vi "_PC_MS_SubVI writeToTDMS.vi"(5 "MS.Pause":refnum<vi>, 7 "warning sign":refnum<vi>, 8 "error in (no error)":errorcluster, 11 "Stop":refnum<vi>) -> (0 "error out":errorcluster)   [LabVIEW 2018]
uses:
  <vilib>/Platform/TimedLoop/XDataNode/timing_clust.ctl
  <vilib>/Platform/TimedLoop/XDataNode/nitl_modes.ctl
  <vilib>/Platform/TimedLoop/XDataNode/wakeup.ctl
  PublicSubVI/Class/FileManager/FM/ctl/_PC_Pub_FM stateMachineEnum.ctl
  PublicSubVI/Class/FileManager/FM/ctl/_PC_Pub_FM ctrlFileRefnumEnum.ctl
  <vilib>/Platform/TimedLoop/XDataNode/XDataNode.xnode
  PublicSubVI/Class/FileManager/FM.lvclass
  <vilib>/Platform/TimedLoop/XDataNode/XDNodeRunTimeDep.lvlib
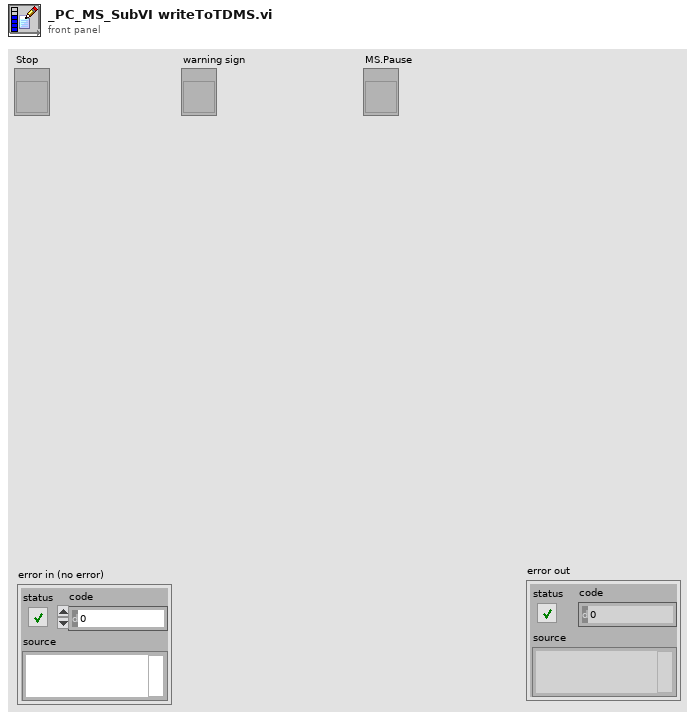
[diagram p1: front panel]
types:
  T1 = typedef "XDNodeRunTimeDep.lvlib/timing_clust.ctl" = cluster{"Expected End [f-1]":u64, "Actual End [f-1]":u64, "Finished Late? [f-1]":bool, "Expected End [i-1]":u64, "Actual End [i-1]":u64, "Finished Late? [i-1]":bool, "Expected Start [i]":u64, "Actual Start [i]":u64, "Expected Start [f]":u64, "Actual Start [f]":u64, "Source Name":string, "Structure Name":string, "Period":i64, "Deadline":i64, "Offset":i64, "Start":i64, "Priority":i32, "Timeout":i32, "Mode":T2, "Wakeup Reason":T3, "Error":errorcluster, "Source Type":string, "Secondary Source Type":string, "Global End Time":u64, "Global Start Time":u64, "Frame Duration":u64, "Iteration Duration":u64, "Assigned CPU":i32, "I/O Scan Engine Mode":u32}
  T2 = typedef "XDNodeRunTimeDep.lvlib/nitl_modes.ctl" = enum32{"No Change", "Process missed periods, maintain original phase", "Discard missed periods, maintain original phase", "Process missed periods, ignore original phase", "Discard missed periods, ignore original phase"}
  T3 = typedef "XDNodeRunTimeDep.lvlib/wakeup.ctl" = enum32{"Normal", "Aborted", "Asynchronous wakeup", "Timing source error", "Timed loop error", "Timeout"}
  T4 = enum16{"None", "Init", "Write", "Read", "PauseRead", "FinishCheck"}
  T5 = typedef "_PC_Pub_FM ctrlFileRefnumEnum.ctl" = enum16{"init", "checkFileName", "updFileName", "updWorkFolder", "updDataItems", "addNewFileName", "addSerialNum"}
  T6 = typedef "_PC_Pub_FM stateMachineEnum.ctl" = enum16{"none", "init", "reset_t0", "openTDMS", "writeTDMS", "closeTDMS", "readTDMS", "getDataItems"}
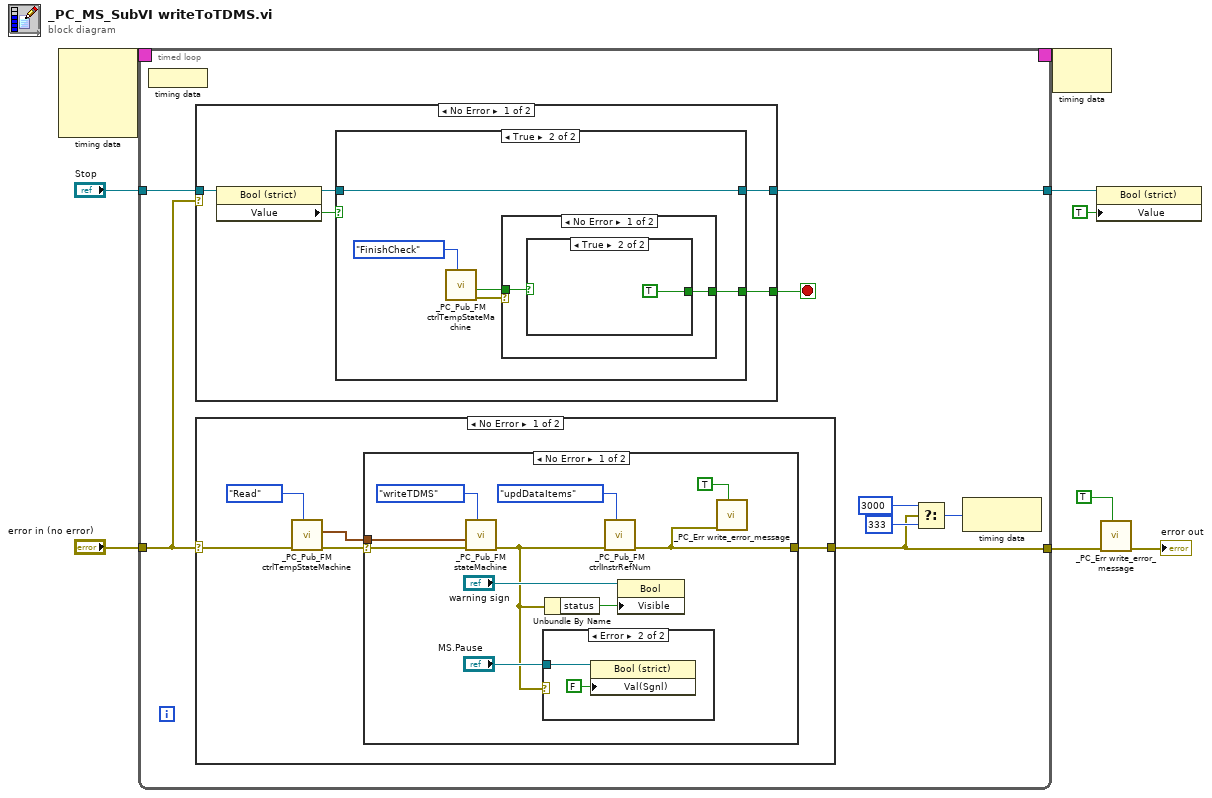
[diagram p0: block diagram]
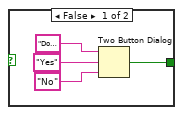
[diagram p3: hidden frame]
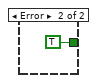
[diagram p4: hidden frame]
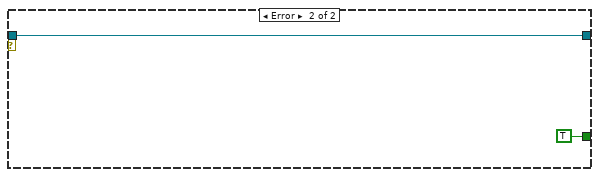
[diagram p5: hidden frame]
diagram:
  n1 = node-c288() -> (w7:T1)  [unwired: 4 in]
  n2 = timed-loop {
    tunnel: "Stop" -> [w12]
    timing: w7 -> [_]
    timing-out: [_] -> w6
    tunnel: "error in (no error)" -> [w13]
    tunnel: [w14] -> w3
    tunnel: [w11] -> w1
    stop <- w10 stop-if-true
    n3 = node-c288() -> ()  [unwired: 1 in]
    n4 = case shown="No Error" w13 {
      tunnel: [w19 TRUE] -> w10
      tunnel: w12 -> [w22 w37]
      tunnel: [w18 w37] -> w11
      frame No Error {
        n5 = property class="Bool (strict)"(reference=w22) -> (reference out=w20:refnum<vi>, "Value"=w21:bool)  [unwired: 1 in, 1 out]
        n6 = case shown="True" w21 {
          tunnel: w20 -> [w23 w24]
          tunnel: [_ w26] -> w19
          tunnel: [w23 w24] -> w18
          frame False {
          }
          frame True {
            n7 = call "_PC_Pub_FM ctrlTempStateMachine.vi"("function"=T4."FinishCheck") -> ("error out"=w25:errorcluster, "finish? (F)"=w27:bool)  [unwired: 8 in, 1 out]
            n8 = case shown="No Error" w25 {
              tunnel: w27 -> [w30 _]
              tunnel: [w29 TRUE ("T button?")] -> w26
              frame No Error {
                n9 = case shown="True" w30 {
                  tunnel: [w33 TRUE] -> w29
                  frame False {
                    n10 = Two Button Dialog(message="Do you want to interrupt this access process?", 1:"No" ("F button name (\"Cancel\")"), 2:"Yes" ("T button name (\"OK\")")) -> (T button?=w33:bool)
                  }
                  frame True {
                  }
                }
              }
              frame Error {
              }
            }
          }
        }
      }
      frame Error {
      }
    }
    n11 = case shown="No Error" w13 {
      selector: w13 -> [w42 w57]
      tunnel: [w43 w57] -> w14
      frame No Error {
        n12 = call "_PC_Pub_FM ctrlTempStateMachine.vi"("function"=T4."Read", "error in (no error)"=w42) -> ("error out"=w40:errorcluster, "outputData"=w41:waveform(sgl))  [unwired: 7 in, 1 out]
        n13 = case shown="No Error" w40 {
          selector: w40 -> [w52 w56]
          tunnel: w41 -> [w45 _]
          tunnel: [w44 w56] -> w43
          frame No Error {
            n14 = call "_PC_Pub_FM stateMachine.vi"("Func"=_PC_Pub_FM_stateMachineEnum."writeTDMS", "error in (no error)"=w52, "elementData"=w45) -> ("error out"=w46:errorcluster)  [unwired: 6 in, 2 out]
            n15 = case shown="Error" w46 {
              tunnel: "MS.Pause" -> [_ w55]
              frame No Error {
              }
              frame Error {
                n16 = property class="Bool (strict)"(reference=w55, "Val(Sgnl)"=FALSE ("Value (Signaling)")) -> ()  [unwired: 1 in, 2 out]
              }
            }
            n17 = Unbundle By Name(w46) -> ("status"=w48:bool)
            n18 = call "_PC_Pub_FM ctrlInstrRefNum.vi"("function"=_PC_Pub_FM_ctrlFileRefnumEnum."updDataItems", "error in (no error)"=w46) -> ("error out"=w44:errorcluster)  [unwired: 9 in]
            n19 = property class="Bool"(reference="warning sign", "Visible"=w48) -> ()  [unwired: 1 in, 2 out]
            n20 = call "_PC_Err write_error_message.vi"("show msg( T )"=TRUE, "error in"=w44) -> ()  [unwired: 9 in, 1 out]
          }
          frame Error {
          }
        }
      }
      frame Error {
      }
    }
    n21 = Select(t=i64 3000, s=w14, f=i64 333) -> (s? t:f=w15:i64)
    n22 = node-c288(w15) -> ()  [unwired: 1 out]
  }
  n23 = node-c288(w6) -> ()  [unwired: 1 out]
  n24 = property class="Bool (strict)"(reference=w1, "Value"=TRUE) -> ()  [unwired: 1 in, 2 out]
  n25 = call "_PC_Err write_error_message.vi"("show msg( T )"=TRUE, "error in"=w3) -> ("error out"=→"error out":errorcluster)  [unwired: 9 in]
